vi "IV_Sweep_multiple_stage_GSM-20H10.vi"(4 "Compliance  Level (A/V)":dbl=0.1, 5 "Delay Time (s)":dbl=1.0, 6 "Source Mode  (0: Voltage)":u16(ring) items=["Voltage", "Current"], 7 "End (mV/uA)":dbl[](array[numeric]), 9 "Writefile":bool=TRUE, 10 "Start(V/mA)":dbl, 11 "Interval (mV/uA)":dbl[](array[numeric])) -> (1 "Resistance":sgl=-680628800000.0, 2 "Current":sgl=-1.469503e-10, 3 "Voltage":sgl=100.0186)   [LabVIEW 2016]
uses:
  <vilib>/Analysis/NI_AALPro.lvlib
  <instrlib>/GSM Series/GSM.lvlib
panel:
  out "intercept":dbl
  out "slope":dbl
  out "Steps (mV/uA)":dbl[](array[numeric])
  in  "Output filename":path
  out "IV":cluster{dbl[], dbl[]}(graph)
  out "VR":cluster{dbl[], dbl[]}(graph)
  out "IR":cluster{dbl[], dbl[]}(graph)
  in  "2wire(F)/4wire(T)":bool
  in  "Enable Resistance Auto Range (T:Enable)":bool=TRUE
  in  "Enable Current Auto Range (T:Enable)":bool=TRUE
  in  "Enable Voltage Auto Range (T:Enable)":bool=TRUE
  in  "Resistance Manual Range (1.0)":dbl=1.0
  in  "Current Manual Range (1.0)":dbl=1.0
  in  "Voltage Manual Range (1.0)":dbl=1.0
  in  "Serial Configuration":T1={"Baud Rate"=9600, "Parity"=0, "Data Bits"=8, "Stop Bits"=10, "Flow Control"=0} {"Flow Control" items=["None", "XON/XOFF", "RTS/CTS", "XON/XOFF & RTS/CTS", "DTR/DSR", "XON/XOFF & DTR/DSR"]; "Stop Bits" items=["1.0"=10, "1.5"=15, "2.0"=20]; "Data Bits" items=["7"=7, "8"=8]; "Parity" items=["None", "Odd", "Even", "Mark", "Space"]; "Baud Rate" items=["300"=300, "600"=600, "1200"=1200, "2400"=2400, "4800"=4800, "9600"=9600, "19200"=19200]}
  in  "VISA resource name":refnum<visa-resource-name>="COM5"
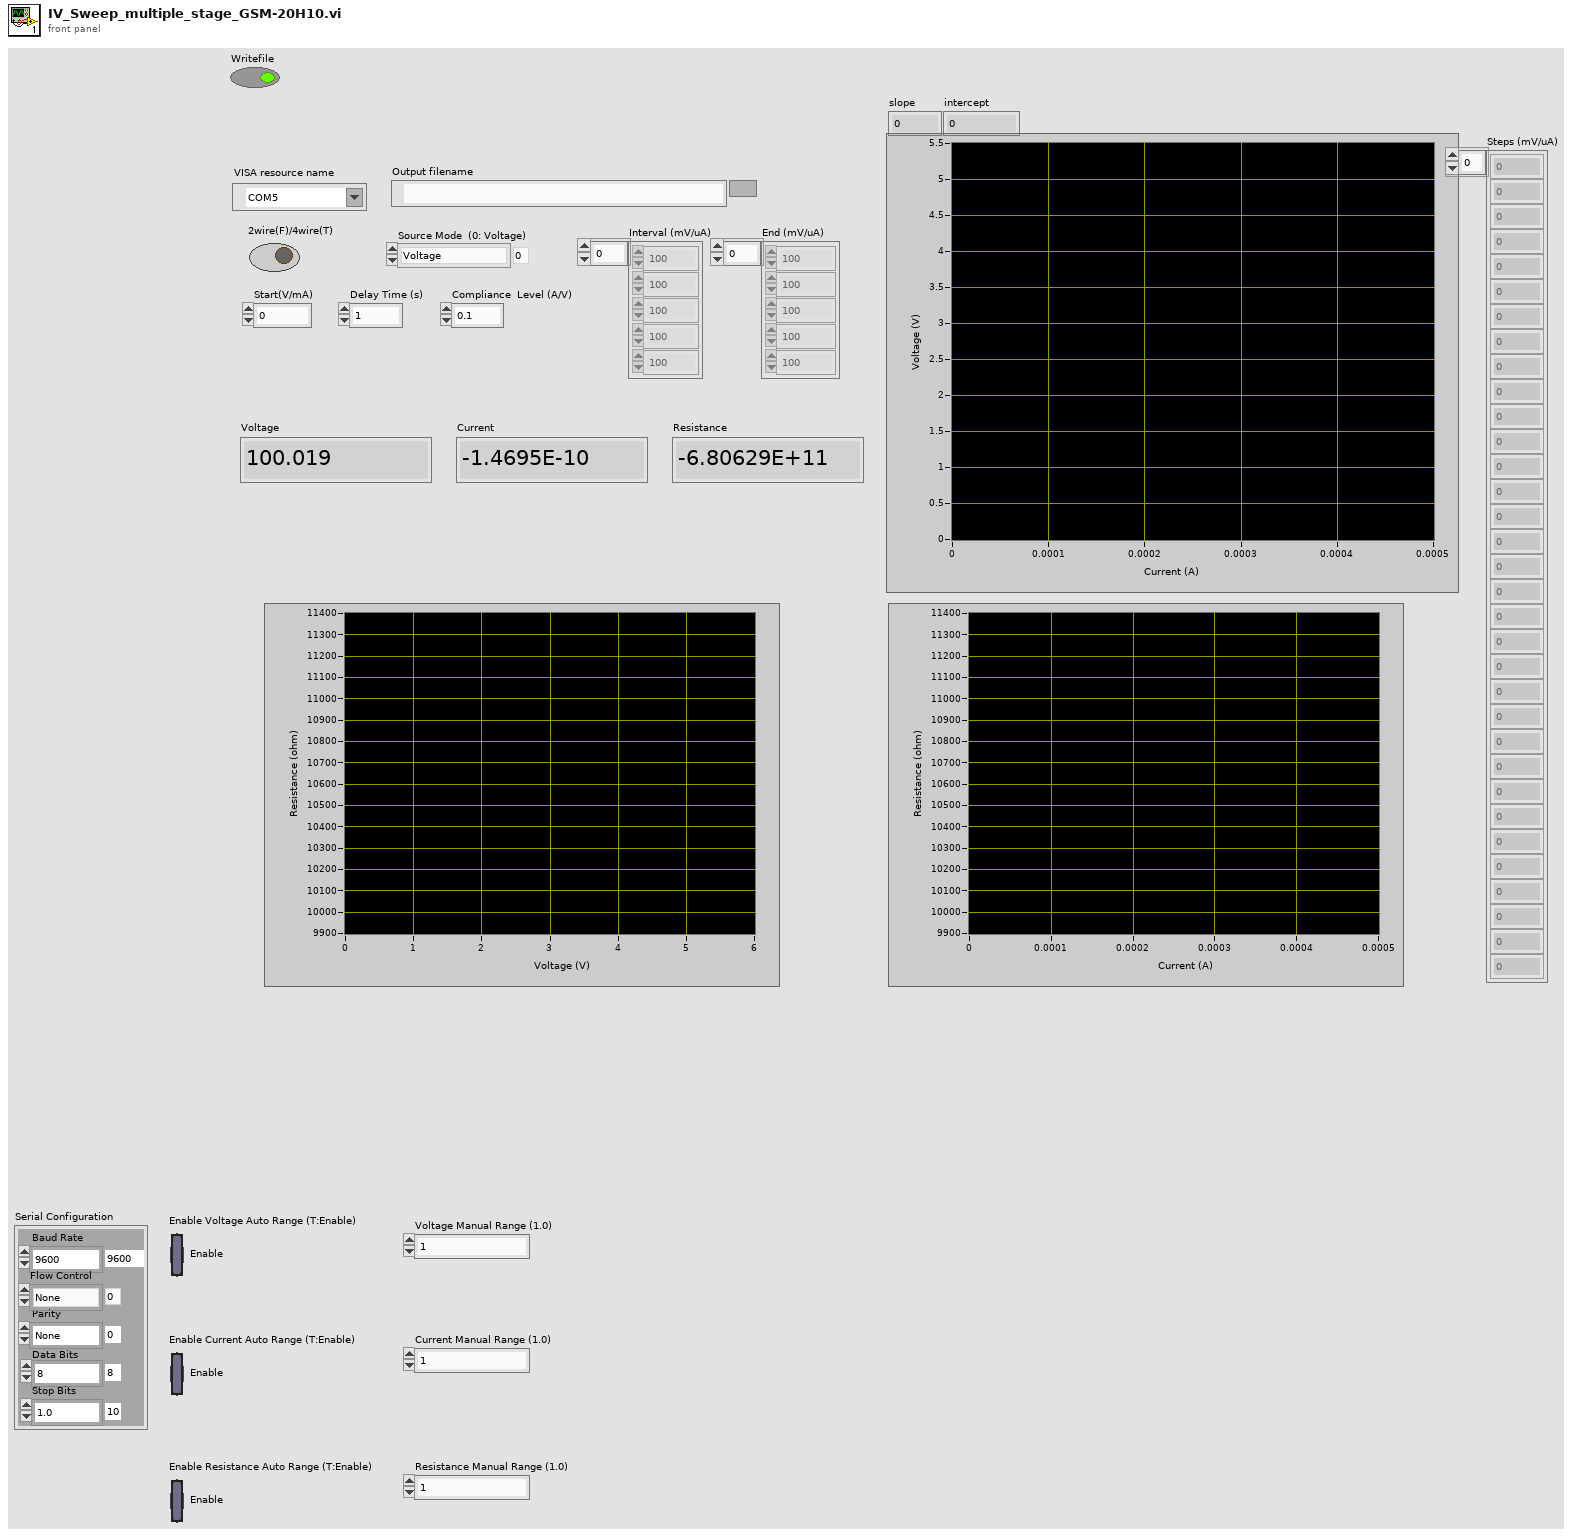
[diagram p1: front panel]
types:
  T1 = cluster{"Baud Rate":u32, "Parity":u16, "Data Bits":u16, "Stop Bits":u16, "Flow Control":u16}
  T2 = enum16{"open", "replace", "create", "open or create", "replace or create", "replace or create with confirmation"}
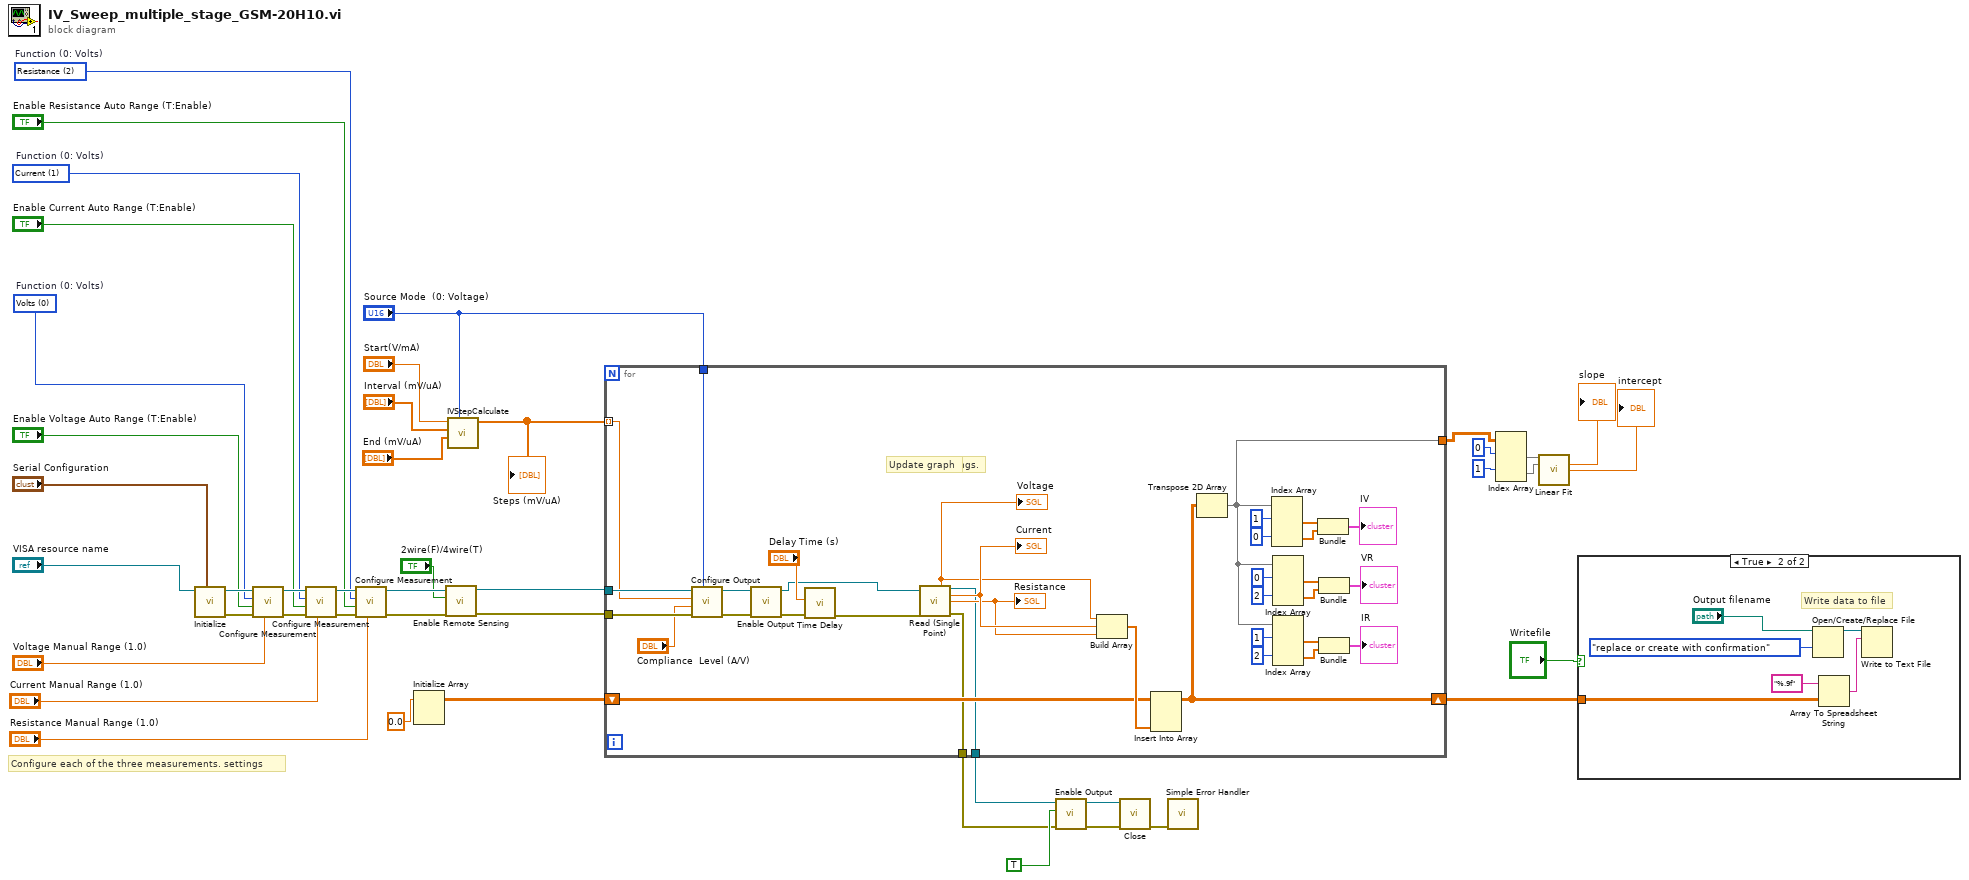
[diagram p0: block diagram]
diagram:
  w34 = u16 2 items=["Volts", "Current", "Resistance"]  # Function (0: Volts)
  w35 = u16 1 items=["Volts", "Current", "Resistance"]  # Function (0: Volts)
  w36 = u16 0 items=["Volts", "Current", "Resistance"]  # Function (0: Volts)
  # "Configure each of the three measurements. settings"
  n1 = call <instrlib>:"Initialize.vi"("Serial Configuration"="Serial Configuration", "VISA resource name"="VISA resource name") -> ("error out"=w41:errorcluster, "VISA resource name out"=w42:refnum<visa-resource-name>)  [unwired: 8 in]
  n2 = call <instrlib>:"Configure Measurement.vi"("Manual Range (1.0)"="Voltage Manual Range (1.0)", "error in (no error)"=w41, "Enable Auto Range (T:Enable)"="Enable Voltage Auto Range (T:Enable)", "Function (0: Volts)"=w36, "VISA resource name"=w42) -> ("error out"=w39:errorcluster, "VISA resource name out"=w40:refnum<visa-resource-name>)  [unwired: 5 in]
  n3 = call <instrlib>:"Configure Measurement.vi"("Manual Range (1.0)"="Current Manual Range (1.0)", "error in (no error)"=w39, "Enable Auto Range (T:Enable)"="Enable Current Auto Range (T:Enable)", "Function (0: Volts)"=w35, "VISA resource name"=w40) -> ("error out"=w38:errorcluster, "VISA resource name out"=w37:refnum<visa-resource-name>)  [unwired: 5 in]
  n4 = call <instrlib>:"Configure Measurement.vi"("Manual Range (1.0)"="Resistance Manual Range (1.0)", "error in (no error)"=w38, "Enable Auto Range (T:Enable)"="Enable Resistance Auto Range (T:Enable)", "Function (0: Volts)"=w34, "VISA resource name"=w37) -> ("error out"=w24:errorcluster, "VISA resource name out"=w25:refnum<visa-resource-name>)  [unwired: 5 in]
  n5 = Initialize Array(0.0 ("element")) -> (w26:dbl[][])  [unwired: 2 in]
  n6 = call <instrlib>:"Enable Remote Sensing.vi"("error in (no error)"=w24, "Enable Remote Sensing (T: Enable)"="2wire(F)/4wire(T)", "VISA resource name"=w25) -> ("error out"=w22:errorcluster, "VISA resource name out"=w23:refnum<visa-resource-name>)  [unwired: 7 in]
  n7 = call "IVStepCalculate.vi"("V(0)/I(1)"="Source Mode  (0: Voltage)", "End"="End (mV/uA)", "Interval"="Interval (mV/uA)", "Start"="Start(V/mA)") -> ("mV/uA"=w17:dbl[])  [unwired: 7 in]
  "Steps (mV/uA)" <- w17
  n8 = for {
    tunnel: w22 -> [w78]
    tunnel: w23 -> [w79]
    shift-right: [w50] -> w16
    shift-left: w26 -> [w54]
    tunnel: w17 -> [w49] mode=indexing
    tunnel: "Source Mode  (0: Voltage)" -> [w48]
    tunnel: [w47] -> w14
    tunnel: [w46] -> w3
    tunnel: [w45] -> w2
    # "Update graph"
    # "Take the readings."
    n9 = call <instrlib>:"Configure Output.vi"("Source Mode  (0: Voltage)"=w48, "error in (no error)"=w78, "Compliance  Level (0.1)"="Compliance  Level (A/V)", "Output Level (0)"=w49, "VISA resource name"=w79) -> ("error out"=w53:errorcluster, "VISA resource name out"=w52:refnum<visa-resource-name>)  [unwired: 5 in]
    n10 = call <instrlib>:"Enable Output.vi"("error in (no error)"=w53, "VISA resource name"=w52) -> ("error out"=w67:errorcluster, "VISA resource name out"=w68:refnum<visa-resource-name>)  [unwired: 8 in]
    n11 = call "Time Delay"("error in (no error)"=w67, "Delay Time (s)"="Delay Time (s)") -> ("error out"=w71:errorcluster)  [unwired: 9 in]
    n12 = call <instrlib>:"Read (Single Point).vi"("VISA resource name"=w68, "error in (no error)"=w71) -> ("Voltage"=w72:sgl, "VISA resource name out"=w46:refnum<visa-resource-name>, "Current"=w73:sgl, "Resistance"=w69:sgl, "error out"=w45:errorcluster)  [unwired: 7 in, 2 out]
    "Voltage" <- w72
    "Current" <- w73
    "Resistance" <- w69
    n13 = Build Array(w72, w73, w69) -> (w74:sgl[])
    n14 = Insert Into Array(array=w54, new element=w74) -> (w50:dbl[][])  [unwired: 2 in]
    n15 = Transpose 2D Array(2D array=w50) -> (transposed array=w47:dbl[][])
    n16 = Index Array(array=w47, index (row) #1=1 ("index (row)"), index (row) #2=0 ("index (row)")) -> (element #1=w76:dbl[], element #2=w77:dbl[])  [unwired: 2 in]
    n17 = Index Array(array=w47, index (row) #1=0 ("index (row)"), index (row) #2=2 ("index (row)")) -> (element #1=w63:dbl[], element #2=w64:dbl[])  [unwired: 2 in]
    n18 = Index Array(array=w47, index (row) #1=1 ("index (row)"), index (row) #2=2 ("index (row)")) -> (element #1=w58:dbl[], element #2=w59:dbl[])  [unwired: 2 in]
    n19 = Bundle(w76, w77) -> (→"IV":cluster{dbl[], dbl[]})  [unwired: 1 in]
    n20 = Bundle(w63, w64) -> (→"VR":cluster{dbl[], dbl[]})  [unwired: 1 in]
    n21 = Bundle(w58, w59) -> (→"IR":cluster{dbl[], dbl[]})  [unwired: 1 in]
  }
  n22 = call <instrlib>:"Enable Output.vi"("error in (no error)"=w2, "Enable Output (T: Enable)"=TRUE, "VISA resource name"=w3) -> ("error out"=w4:errorcluster, "VISA resource name out"=w5:refnum<visa-resource-name>)  [unwired: 7 in]
  n23 = call <instrlib>:"Close.vi"("error in (no error)"=w4, "VISA resource name"=w5) -> ("error out"=w7:errorcluster)  [unwired: 9 in]
  n24 = call <vilib>:"Simple Error Handler.vi"("error in (no error)"=w7) -> ()  [unwired: 4 in, 5 out]
  n25 = Index Array(array=w14, index (row) #1=0 ("index (page)"), index (row) #2=1 ("index (row)")) -> (element #1=w11:dbl[], element #2=w10:dbl[])  [unwired: 2 in]
  n26 = call <vilib>:"Linear Fit.vi"("Y"=w11, "X"=w10) -> ("slope"=→"slope":dbl, "intercept"=→"intercept":dbl)  [unwired: 9 in, 3 out]
  n27 = case shown="True" "Writefile" {
    tunnel: w16 -> [_ w80]
    frame False {
    }
    frame True {
      # "Write data to file"
      n28 = Open/Create/Replace File(file path (use dialog)="Output filename", operation (0:open)=T2."replace or create with confirmation") -> (refnum out=w84:refnum<file>)  [unwired: 4 in, 2 out]
      n29 = Array To Spreadsheet String(array=w80, 3:"%.9f" ("format string")) -> (spreadsheet string=w81:string)  [unwired: 1 in]
      n30 = Write to Text File(file (use dialog)=w84, text=w81) -> ()  [unwired: 2 in, 3 out]
    }
  }
